vi "Error Sound.vi"   [LabVIEW 2020, in "SubVIs.lvlib"]
uses:
  SubVIs.lvlib
types:
  T1 = typedef "Sound Output Task ID.ctl" = u32
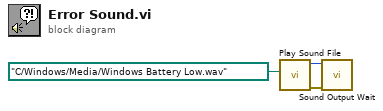
[diagram p0: block diagram]
diagram:
  n1 = call <vilib>:"Play Sound File.vi"("path"=path "C:/Windows/Media/Windows Battery Low.wav") -> ("error out"=w1:errorcluster, "task ID"=w2:T1)  [unwired: 9 in]
  n2 = call <vilib>:"Sound Output Wait.vi"("error in (no error)"=w1, "task ID"=w2) -> ()  [unwired: 8 in, 2 out]
